vi "Define Suite.vi"(5 "Banana Peels":refnum<class "BananaPeel.lvclass">[](array[class]), 7 "Test Report (optional)":refnum<class "Test Report.lvclass">, 8 "error in":errorcluster, 10 "Interactive":bool, 11 "Label (VI Title)":string) -> (0 "error out":errorcluster, 2 "Properties.Suite":refnum<class "Properties.Suite.lvclass">, 3 "Platano":refnum<class "Platano.CarayaTestSuite.lvclass">)   [LabVIEW 2021, in "Banana.Caraya.lvlib" / "Platano.CarayaTestSuite.lvclass"]
uses:
  Platano.CarayaTestSuite.lvclass
  <vilib>/addons/_JKI Toolkits/Caraya/classes/Properties.Suite/Properties.Suite.lvclass
  C:/Repositories/LVOS/Bananas/lv-src/Bananas/Platano/Platano.lvclass
  <vilib>/addons/_JKI Toolkits/Caraya/classes/Test Report/Test Report.lvclass
  Bananas/BananaPeel/BananaPeel.lvclass
  Bananas/Banana/Banana.lvclass/Banana.ctl
  Bananas/DefineSuite/DefineSuite.lvclass/DefineSuite.ctl
  Bananas/DefineSuite/Write Interactive.vi
  <vilib>/LabVIEW Open Source Project/Data Manipulation/Variant/Variant_SetName.vi
  <vilib>/LabVIEW Open Source Project/Data Manipulation/Variant/Variant_BuildClusterFromElementArray.vi
  Bananas/Banana/Read Ephemerals.vi
  <vilib>/LabVIEW Open Source Project/Data Manipulation/Variant/Variant_EmptyCluster.vi
  Bananas/DefineSuite/DefineSuite.lvclass
  C:/Repositories/LVOS/Bananas/lv-src/Bananas/BananaPeel/BananaPeel.lvclass
  Leaf.Properties.Suite/Leaf.Properties.Suite.lvclass
  C:/Repositories/LVOS/Bananas/lv-src/Bananas/Leaf.TestSuite/Leaf.TestSuite.lvclass
  <vilib>/addons/_JKI Toolkits/Caraya/classes/Test Suite/Define Test Suite (Default).vi
  <vilib>/LabVIEW Open Source Project/Data Manipulation/Variant/Variant_ListElements.vi
  <vilib>/LabVIEW Open Source Project/Data Manipulation/TypeDescriptor/TypeDescriptor_SetName.vi
  <vilib>/Utility/GetType.llb/TD_Create Cluster.vi
  Bananas/DefineTest/DefineTest.lvclass
  Bananas/DestroySuite/DestroySuite.lvclass
  Platano.CarayaTestSuite.lvclass/Platano.CarayaTestSuite.ctl
  Bananas/Banana/Banana.lvclass
  Bananas/Platano/Platano.lvclass
  <vilib>/addons/_JKI Toolkits/Caraya/classes/Test Suite/Test Suite.lvclass
  C:/Repositories/LVOS/Bananas/lv-src/Banana.Caraya/Platano.CarayaTestSuite/Platano.CarayaTestSuite.lvclass
  C:/Repositories/LVOS/Bananas/lv-src/Bananas/DefineSuite/DefineSuite.lvclass
  C:/Repositories/LVOS/Bananas/lv-src/Banana.Caraya/Leaf.Properties/Leaf.Properties.lvclass
  C:/Program Files (x86)/National Instruments/LabVIEW 2021/vi.lib/addons/_JKI Toolkits/Caraya/classes/Properties/Properties.lvclass
  C:/Repositories/LVOS/Bananas/lv-src/Bananas/Leaf/Leaf.lvclass
  C:/Repositories/LVOS/Bananas/lv-src/Banana.Caraya/Leaf.Properties.Suite/Leaf.Properties.Suite.lvclass
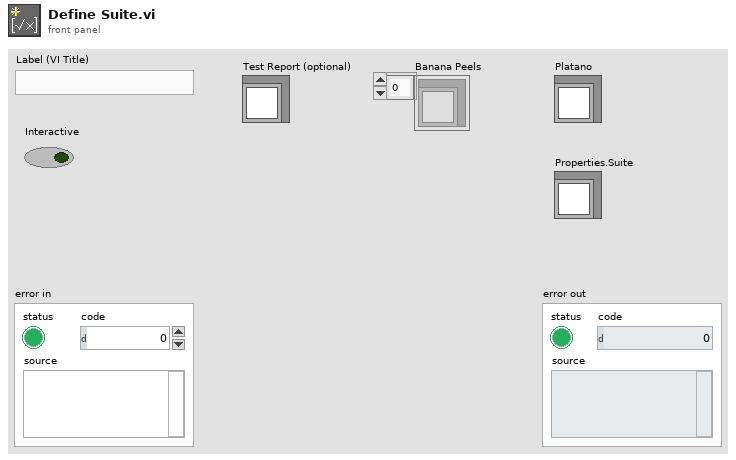
[diagram p1: front panel]
types:
  T1 = typedef "Bananas.lvlib/Test Strategies -- cluster.ctl" = cluster{"DefineTest":refnum<class "DefineTest.lvclass">, "DefineSuite":refnum<class "DefineSuite.lvclass">, "DestroySuite":refnum<class "DestroySuite.lvclass">}
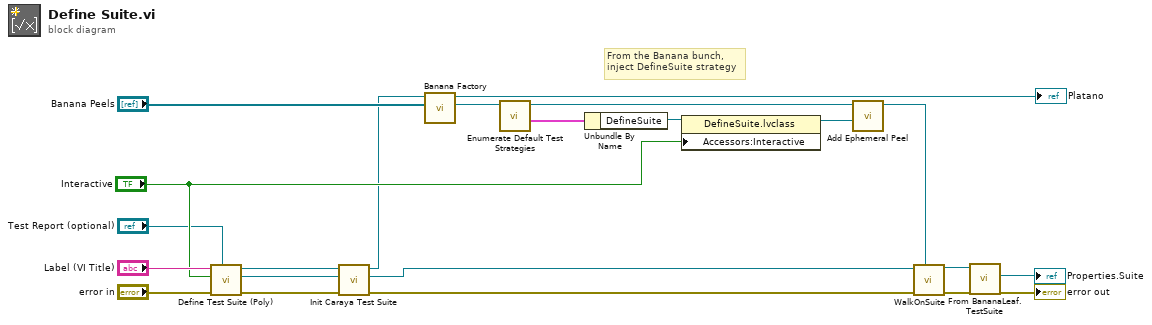
[diagram p0: block diagram]
diagram:
  # "From the Banana bunch,\ninject DefineSuite strategy"
  n1 = call-poly <vilib>:"Define Test Suite (Poly).vi"("Test Report (optional)"="Test Report (optional)", "error in (no error)"="error in", "Interactive"="Interactive", "Label (VI Title)"="Label (VI Title)") -> ("error out"=w11:errorcluster, "Properties.Suite"=w1:refnum<class "Properties.Suite.lvclass">, "Test Suite"=w13:refnum<class "Test Suite.lvclass">)  [unwired: 5 in]
  n2 = call "Init Caraya Test Suite.vi"("error in (no error)"=w11, "Properties.Suite"=w1, "TestSuite"=w13) -> ("error out"=w10:errorcluster, "Leaf.Properties.TestSuite out"=w4:refnum<class "Leaf.Properties.Suite.lvclass">, "Platano.CarayaTestSuite out"=w5:refnum<class "Platano.CarayaTestSuite.lvclass">)  [unwired: 6 in]
  n3 = call "Banana Factory.vi"("Peels"="Banana Peels", "Platano"=w5) -> ("Banana"=w7:refnum<class "Banana.lvclass">, "Platano dup"=→"Platano":refnum<class "Platano.CarayaTestSuite.lvclass">)  [unwired: 8 in]
  n4 = call "Enumerate Default Test Strategies.vi"("Banana"=w7) -> ("Strategies"=w21:T1, "Banana"=w20:refnum<class "Banana.lvclass">)  [unwired: 9 in]
  n5 = Unbundle By Name(w21) -> ("DefineSuite"=w16:refnum<class "DefineSuite.lvclass">)
  n6 = property class="DefineSuite.lvclass"(reference=w16, "Accessors:Interactive"="Interactive") -> (reference out=w15:refnum<class "DefineSuite.lvclass">)  [unwired: 1 in, 1 out]
  n7 = call "Add Ephemeral Peel.vi"("BananaPeel"=w15, "Banana"=w20) -> ("Banana"=w12:refnum<class "Banana.lvclass">)  [unwired: 9 in]
  n8 = call "WalkOnSuite.vi"("Banana"=w12, "error in (no error)"=w10, "Leaf.TestSuite"=w4) -> ("error out"=→"error out":errorcluster, "Leaf.TestSuite"=w3:refnum<class "Leaf.Properties.Suite.lvclass">)  [unwired: 7 in]
  n9 = call "From BananaLeaf.TestSuite.vi"("Leaf.Properties.TestSuite"=w3) -> ("Properties.Suite"=→"Properties.Suite":refnum<class "Properties.Suite.lvclass">)  [unwired: 10 in]
